vi "PathPlanner_Trajectory_Sample.vi"(9 "Time":dbl, 11 "PathPlannerTrajectory":T5 {"States"."TargetHolonomicRotation"."SIN" format="%13.4f"; "States"."TargetHolonomicRotation"."COS" format="%13.4f"; "States"."TargetHolonomicRotation"."VALUE" format="%13.4f"; "States"."Heading"."SIN" format="%13.4f"; "States"."Heading"."COS" format="%13.4f"; "States"."Heading"."VALUE" format="%13.4f"; "States"."PositionMeters"."Y" format="%14.3f"; "States"."PositionMeters"."X" format="%14.3f"}) -> (3 "PathPlannerState":T1={"TimeSeconds"=0.0, "VelocityMPS"=0.0, "AccerationMpsSq"=0.0, "HeadingAngularVelRadPerSec"=0.0, "PositionMeters"={"X"=0.0, "Y"=1.0}, "Heading"={"VALUE"=0.0, "COS"=1.0, "SIN"=0.0}, "TargetHolonomicRotation"={"VALUE"=0.0, "COS"=1.0, "SIN"=0.0}, "CurvatureRadPerMeter"=0.0, "PathPlannerConstraints"={"MaxVelocityMps;"=0.0, "MaxAccelerationMpsSq;"=0.0, "MaxAngularVelRadPsEc;"=0.0, "MaxAngularAccRadPSecSq"=0.0, "Exists"=FALSE}, "DeltaPos"=0.0} {"TargetHolonomicRotation"."SIN" format="%13.4f"; "TargetHolonomicRotation"."COS" format="%13.4f"; "TargetHolonomicRotation"."VALUE" format="%13.4f"; "Heading"."SIN" format="%13.4f"; "Heading"."COS" format="%13.4f"; "Heading"."VALUE" format="%13.4f"; "PositionMeters"."Y" format="%14.3f"; "PositionMeters"."X" format="%14.3f"})   [LabVIEW 2019, in "PathPlanner24.lvlib"]
doc: "Get the target state at the given point in time along the trajectory\n\nInputs:\n -- PathPlannerTraectory -- trajectory - PathPlanner Trajectory data cluster\n -- time -- double - The time to sample\n\nOutputs:\n - PathPlannerState - trajectorystate - The state at the given point in time"
uses:
  PathPlanner24.lvlib
  TypeDef/PathPlannerTrajectory.ctl
  TypeDef/PathPlannerTrajectoryState.ctl
  <vilib>/Rock Robotics/WPI/ThirdParty/JAS_Junk/TrajLib/TypeDef/TRANSLATION2D.ctl
  <vilib>/Rock Robotics/WPI/ThirdParty/JAS_Junk/TrajLib/TypeDef/ROTATION2D.ctl
  TypeDef/PathPlannerPathConstraints.ctl
  <vilib>/Rock Robotics/WPI/ThirdParty/JAS_Junk/TrajLib/Trajectory_Library.lvlib
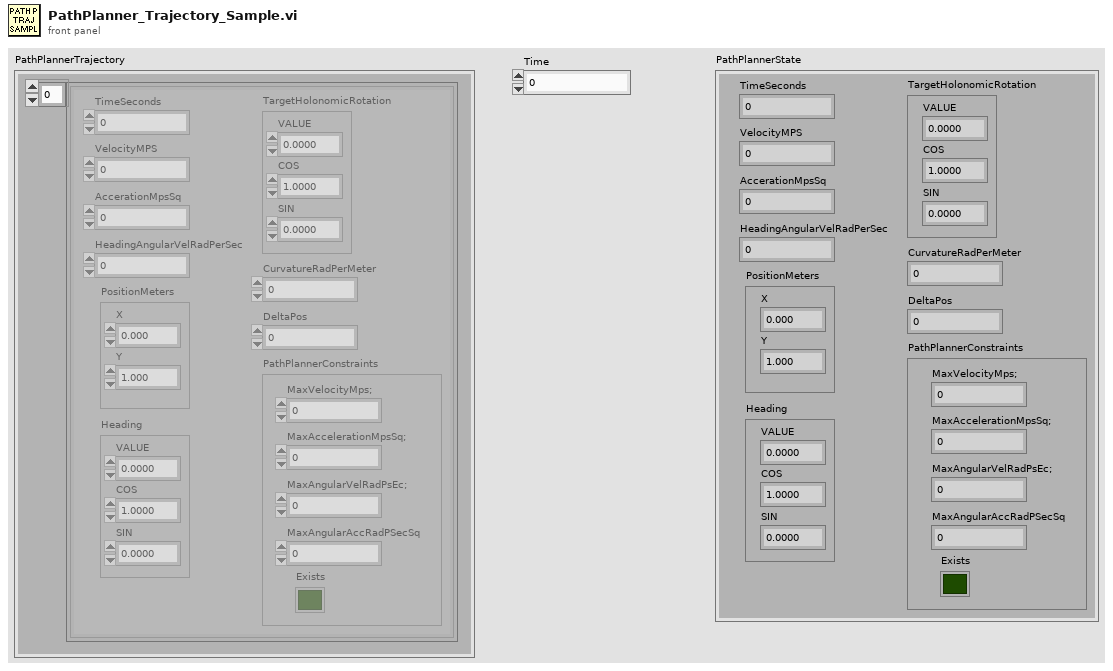
[diagram p1: front panel]
types:
  T1 = typedef "PathPlanner24.lvlib/PathPlannerTrajectoryState.ctl" = cluster{"TimeSeconds":dbl, "VelocityMPS":dbl, "AccerationMpsSq":dbl, "HeadingAngularVelRadPerSec":dbl, "PositionMeters":T2, "Heading":T3, "TargetHolonomicRotation":T3, "CurvatureRadPerMeter":dbl, "PathPlannerConstraints":T4, "DeltaPos":dbl}
  T2 = typedef "Trajectory_Library.lvlib/TRANSLATION2D.ctl" = cluster{"X":dbl, "Y":dbl}
  T3 = typedef "Trajectory_Library.lvlib/ROTATION2D.ctl" = cluster{"VALUE":dbl, "COS":dbl, "SIN":dbl}
  T4 = typedef "PathPlanner24.lvlib/PathPlannerPathConstraints.ctl" = cluster{"MaxVelocityMps;":dbl, "MaxAccelerationMpsSq;":dbl, "MaxAngularVelRadPsEc;":dbl, "MaxAngularAccRadPSecSq":dbl, "Exists":bool}
  T5 = typedef "PathPlanner24.lvlib/PathPlannerTrajectory.ctl" = cluster{"States":T1[]}
  T6 = typedef "PathPlanner.lvlib/PathPlannerTrajectoryState.ctl" = cluster{"TimeSeconds":dbl, "VelocityMPS":dbl, "AccerationMpsSq":dbl, "HeadingAngularVelRadPerSec":dbl, "PositionMeters":T2, "Heading":T3, "TargetHolonomicRotation":T3, "CurvatureRadPerMeter":dbl, "PathPlannerConstraints":T7, "DeltaPos":dbl}
  T7 = typedef "PathPlanner.lvlib/PathPlannerPathConstraints.ctl" = cluster{"MaxVelocityMps;":dbl, "MaxAccelerationMpsSq;":dbl, "MaxAngularVelRadPsEc;":dbl, "MaxAngularAccRadPSecSq":dbl, "Exists":bool}
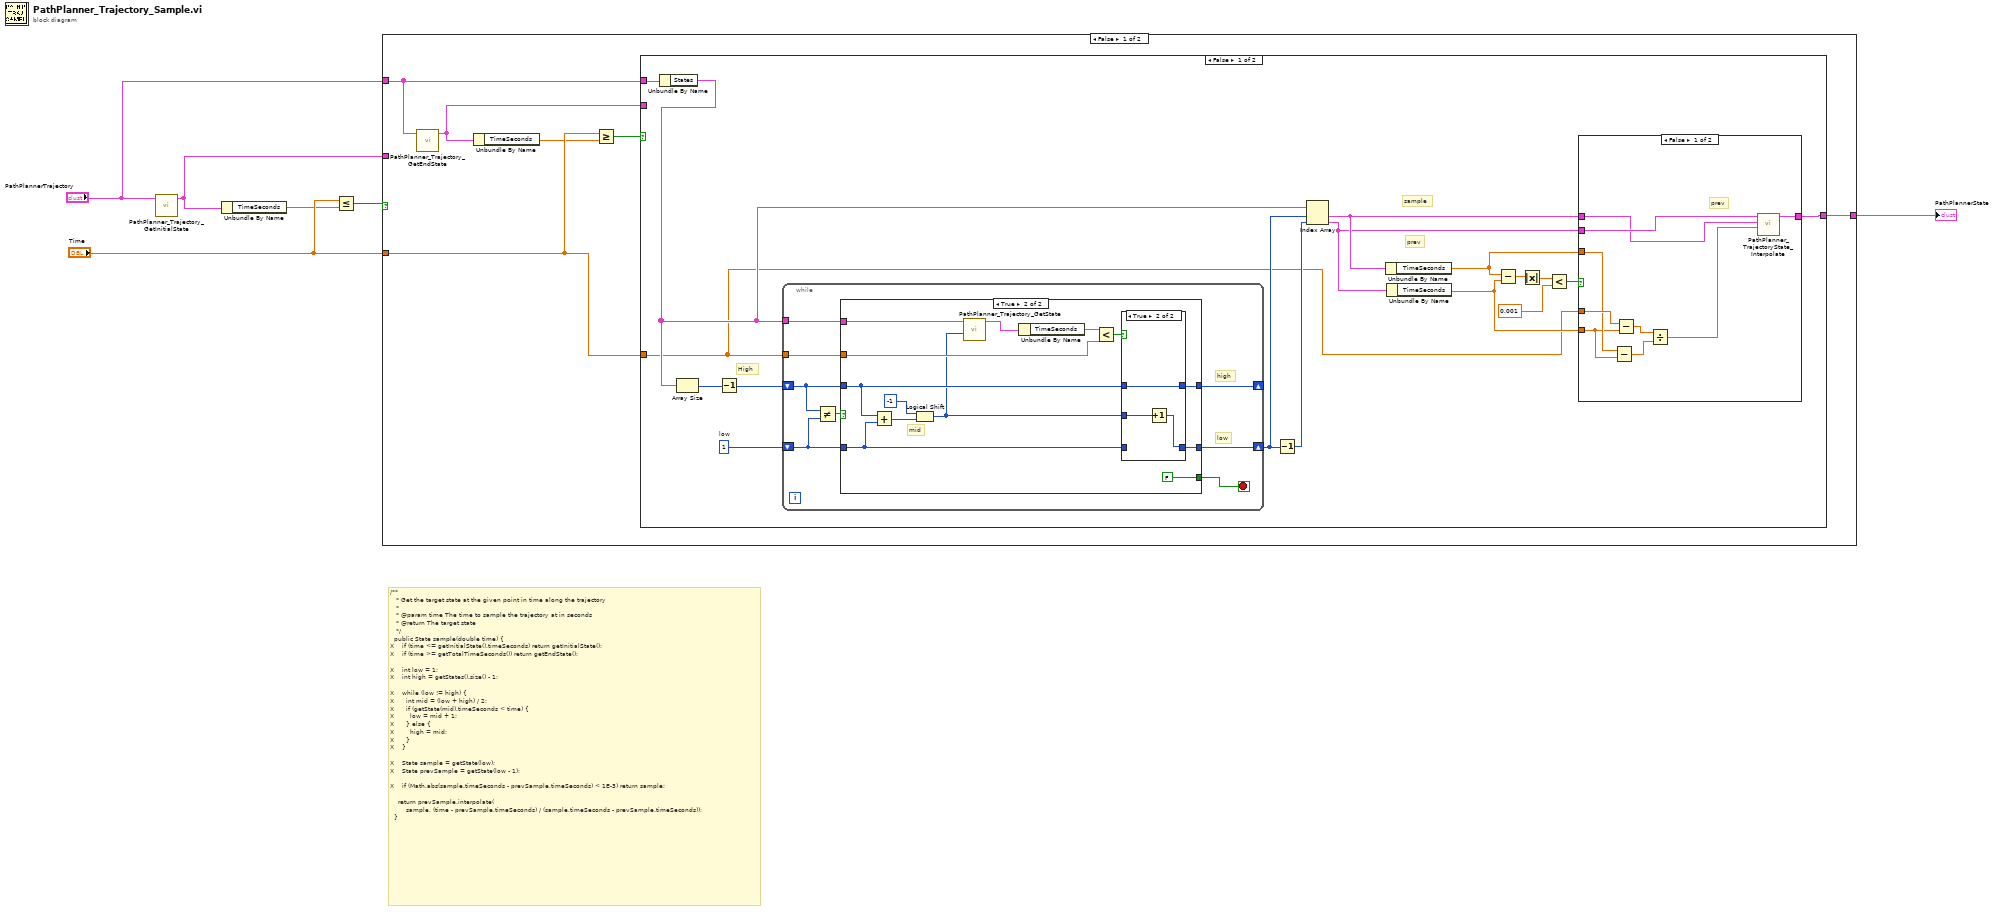
[diagram p0: block diagram]
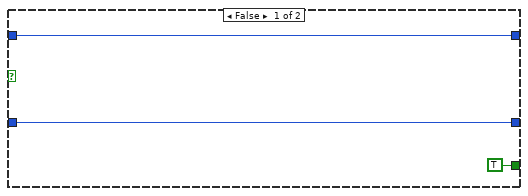
[diagram p3: hidden frame]
diagram:
  # "/**\n   * Get the target state at the given point in time along the trajectory\n   *\n   * @param time The time to sample the trajectory at in seconds\n   * @return The target state\n   */\n  public State sample(double time) {\nX    if (time <= getInitialState().timeSeconds) return getInitialState();\nX    if (time >= getTotalTimeSeconds()) return getEndState();\n\nX    int low = 1;\nX    int high = getStates().size() - 1;\n\nX    while (low != high) {\nX      int mid = (low + high) / 2;\nX      if (getState(mid).timeSeconds < time) {\nX        low = mid + 1;\nX      } else {\nX        high = mid;\nX      }\nX    }\n\nX    State sample = getState(low);\nX    State prevSample = getState(low - 1);\n\nX    if (Math.abs(sample.timeSeconds - prevSample.timeSeconds) < 1E-3) return sample;\n\n    return prevSample.interpolate(\n        sample, (time - prevSample.timeSeconds) / (sample.timeSeconds - prevSample.timeSeconds));\n  }"
  n1 = call "PathPlanner_Trajectory_GetInitialState.vi"("PathPlannerTrajectory"="PathPlannerTrajectory") -> ("PathPlannerState"=w5:T6)  [unwired: 10 in]
  n2 = Unbundle By Name(w5) -> ("TimeSeconds"=w1:dbl)
  n3 = Less Or Equal?(x="Time", y=w1) -> (x <= y?=w6:bool)
  n4 = case shown="False" w6 {
    tunnel: w5 -> [_ w70]
    tunnel: [w10 w70] -> w3
    tunnel: "PathPlannerTrajectory" -> [w9 _]
    tunnel: "Time" -> [w8 _]
    frame False {
      n5 = call "PathPlanner_Trajectory_GetEndState.vi"("PathPlannerTrajectory"=w9) -> ("EndState"=w11:T1)  [unwired: 10 in]
      n6 = Unbundle By Name(w11) -> ("TimeSeconds"=w7:dbl)
      n7 = Greater Or Equal?(x=w8, y=w7) -> (x >= y?=w12:bool)
      n8 = case shown="False" w12 {
        tunnel: w11 -> [_ w69]
        tunnel: [w17 w69] -> w10
        tunnel: w9 -> [w29 _]
        tunnel: w8 -> [w14 _]
        frame False {
          w26 = 1  # low
          # "prev"
          # "sample"
          # "High"
          n9 = Unbundle By Name(w29) -> ("States"=w25:T1[])
          n10 = Array Size(array=w25) -> (size(s)=w28:i32)
          n11 = Decrement(x=w28) -> (x-1=w27:i32)
          n12 = while {
            shift-right: [w45] -> w24
            shift-left: w26 -> [w41]
            shift-right: [w46] -> _
            shift-left: w27 -> [w42]
            tunnel: w25 -> [w44]
            tunnel: w14 -> [w47]
            stop <- w40 stop-if-true
            # "high"
            # "low"
            n13 = Not Equal?(x=w42, y=w41) -> (x != y?=w43:bool)
            n14 = case shown="True" w43 {
              tunnel: w47 -> [_ w60]
              tunnel: w42 -> [w50 w58]
              tunnel: w41 -> [w49 w57]
              tunnel: [w50 w56] -> w46
              tunnel: [w49 w55] -> w45
              tunnel: w44 -> [_ w52]
              tunnel: [TRUE FALSE] -> w40
              frame False {
              }
              frame True {
                # "mid"
                n15 = Add(x=w58, y=w57) -> (x+y=w63:i32)
                n16 = Logical Shift(y=i16 -1, x=w63) -> (x << y=w54:i32)
                n17 = call "PathPlanner_Trajectory_GetState.vi"("index"=w54, "PathPlannerStates"=w52) -> ("PathPlannerState"=w53:T1)  [unwired: 9 in]
                n18 = Unbundle By Name(w53) -> ("TimeSeconds"=w61:dbl)
                n19 = Less?(x=w61, y=w60) -> (x < y?=w59:bool)
                n20 = case shown="True" w59 {
                  tunnel: w58 -> [_ w68]
                  tunnel: [w64 w68] -> w56
                  tunnel: w54 -> [w64 w67]
                  tunnel: w57 -> [w65 _]
                  tunnel: [w65 w66] -> w55
                  frame False {
                  }
                  frame True {
                    n21 = Increment(x=w67) -> (x+1=w66:i32)
                  }
                }
              }
            }
          }
          n22 = Decrement(x=w24) -> (x-1=w23:i32)
          n23 = Index Array(array=w25, index #1=w24, index #2=w23) -> (element #1=w18:T1, element #2=w16:T1)
          n24 = Unbundle By Name(w18) -> ("TimeSeconds"=w13:dbl)
          n25 = Unbundle By Name(w16) -> ("TimeSeconds"=w15:dbl)
          n26 = Subtract(x=w13, y=w15) -> (x-y=w22:dbl)
          n27 = Absolute Value(x=w22) -> (abs(x)=w21:dbl)
          n28 = Less?(x=w21, y=0.001) -> (x < y?=w19:bool)
          n29 = case shown="False" w19 {
            tunnel: w18 -> [w31 w39]
            tunnel: [w38 w39] -> w17
            tunnel: w16 -> [w32 _]
            tunnel: w15 -> [w35 _]
            tunnel: w14 -> [w37 _]
            tunnel: w13 -> [w36 _]
            frame False {
              # "prev"
              n30 = Subtract(x=w36, y=w35) -> (x-y=w33:dbl)
              n31 = Subtract(x=w37, y=w35) -> (x-y=w34:dbl)
              n32 = Divide(x=w34, y=w33) -> (x/y=w30:dbl)
              n33 = call "PathPlanner_TrajectoryState_Interpolate.vi"("Time"=w30, "end Val"=w31, "in PathPlannerState"=w32) -> ("interpolated PathPlanner State"=w38:T1)  [unwired: 8 in]
            }
            frame True {
            }
          }
        }
        frame True {
        }
      }
    }
    frame True {
    }
  }
  "PathPlannerState" <- w3
